vi "cursor_copy.vi"(7 "xy_graph_reference":refnum<vi>, 8 "error in (no error)":errorcluster, 11 "active_curosr":u32) -> (0 "error out":errorcluster, 3 "cursor_configuration":T1)   [LabVIEW 2015, in "lv-graph.lvlib"]
doc: "This VI can be used to copy the configuration of a given cursor indexed by active_cursor."
uses:
  lv-graph.lvlib
  _controls/configuration_cursor.ctl
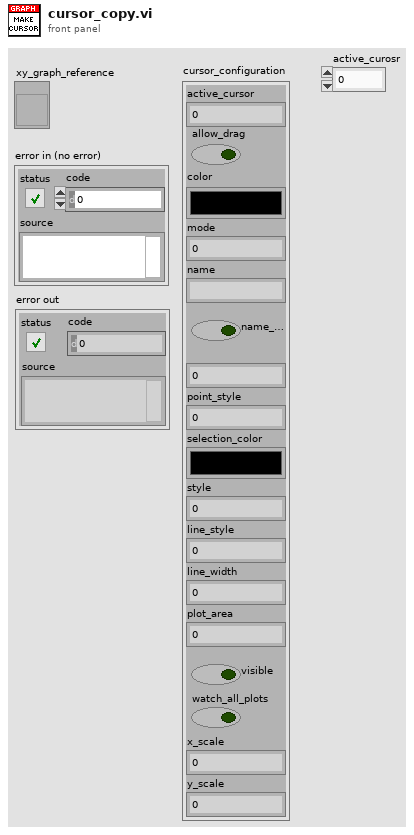
[diagram p1: front panel]
types:
  T1 = typedef "lv-graph.lvlib/configuration_cursor.ctl" = cluster{"active_cursor":u32, "allow_drag":bool, "color":u32, "mode":u32, "name":string, "name_visible":bool, "cursor_plot":i32, "point_style":u8, "selection_color":u32, "style":u8, "line_style":u8, "line_width":u8, "plot_area":i32, "visible":bool, "watch_all_plots":bool, "x_scale":u32, "y_scale":u32}
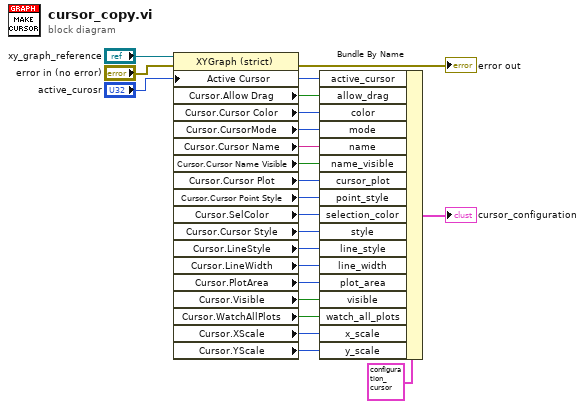
[diagram p0: block diagram]
diagram:
  n1 = property class="XYGraph (strict)"(reference="xy_graph_reference", error in="error in (no error)", "Active Cursor"="active_curosr") -> (error out=→"error out":errorcluster, "Cursor.Allow Drag"=w16:bool, "Cursor.Cursor Color"=w15:u32, "Cursor.CursorMode"=w14:u32, "Cursor.Cursor Name"=w12:string, "Cursor.Cursor Name Visible"=w13:bool, "Cursor.Cursor Plot"=w11:i32, "Cursor.Cursor Point Style"=w10:u8, "Cursor.SelColor"=w9:u32, "Cursor.Cursor Style"=w8:u8, "Cursor.LineStyle"=w7:u8, "Cursor.LineWidth"=w6:u8, "Cursor.PlotArea"=w5:i32, "Cursor.Visible"=w4:bool, "Cursor.WatchAllPlots"=w3:bool, "Cursor.XScale"=w2:u32, "Cursor.YScale"=w1:u32)  [unwired: 1 out]
  n2 = Bundle By Name(cluster=T1 {"active_cursor"=0, "allow_drag"=FALSE, "color"=0, "mode"=0, "name"="", "name_visible"=FALSE, "cursor_plot"=0, "point_style"=0, "selection_color"=0, "style"=0, "line_style"=0, "line_width"=0, "plot_area"=0, "visible"=FALSE, "watch_all_plots"=FALSE, "x_scale"=0, "y_scale"=0} ("cursor_configuration"), "active_cursor"="active_curosr", "allow_drag"=w16, "color"=w15, "mode"=w14, "name"=w12, "name_visible"=w13, "cursor_plot"=w11, "point_style"=w10, "selection_color"=w9, "style"=w8, "line_style"=w7, "line_width"=w6, "plot_area"=w5, "visible"=w4, "watch_all_plots"=w3, "x_scale"=w2, "y_scale"=w1) -> (→"cursor_configuration":T1)
